vi "04. Streaming Simulator.vi"(8 "error in":errorcluster, 10 "request":T1, 11 "Actor Class":T2) -> (0 "error out":errorcluster)   [LabVIEW 2019]
uses:
  Actor/Actor Private Data.ctl
  <vilib>/LabVIEW Open Source Project/MQTT Client/Client class/Client.lvclass
  Actor/Actor Private Events -- cluster.ctl
  Actor/Payload -- cluster.ctl
  streaming-request -- cluster.ctl
  <vilib>/LabVIEW Open Source Project/OpenURI/uri/URI.lvclass/URI.ctl
  <vilib>/LabVIEW Open Source Project/OpenURI/uri/URI.lvclass
panel:
  out "Download Progress":dbl(slide) scale=0.0..100.0
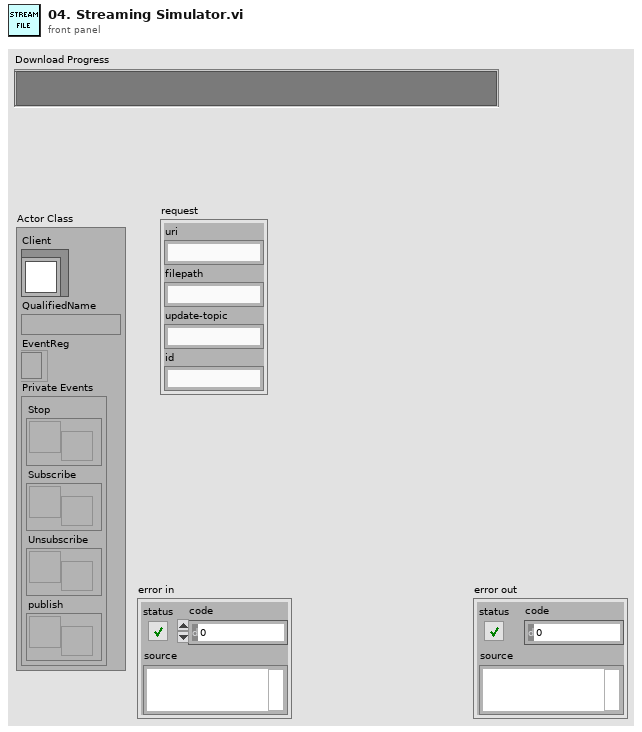
[diagram p1: front panel]
types:
  T1 = typedef "streaming-request -- cluster.ctl" = cluster{"uri":string, "filepath":string, "update-topic":string, "id":string}
  T2 = typedef "Actor Private Data.ctl" = cluster{"Client":refnum<class "Client.lvclass">, "QualifiedName":string, "EventReg":refnum<event-registration>, "Private Events":T3}
  T3 = typedef "Actor Private Events -- cluster.ctl" = cluster{"Stop":refnum<user-event>, "Subscribe":refnum<user-event>, "Unsubscribe":refnum<user-event>, "publish":refnum<user-event>}
  T4 = cluster{"progress (%)":dbl, "complete":bool, "error":bool}
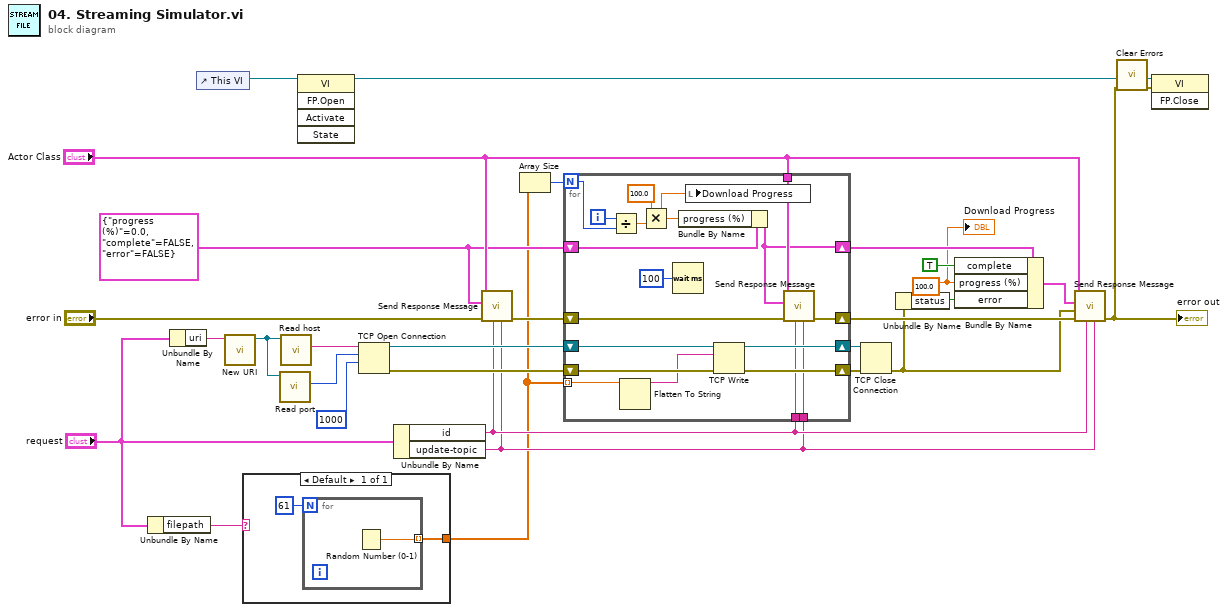
[diagram p0: block diagram]
diagram:
  w4 = 100.0 ("x")
  w26 = T4 {"progress (%)"=0.0, "complete"=FALSE, "error"=FALSE}
  n1 = Unbundle By Name("request") -> ("filepath"=w12:string)
  n2 = Unbundle By Name("request") -> ("uri"=w23:string)
  n3 = control-ref of="This VI"() -> (w5:refnum<vi>)
  n4 = call <vilib>:"New URI.vi"("URI"=w23) -> ("URI"=w21:refnum<class "URI.lvclass">)  [unwired: 9 in, 1 out]
  n5 = case shown="Default" w12 {
    tunnel: [w31] -> w10
    frame Default {
      n6 = for {
        N: 61 ("dimension size") -> [_]
        tunnel: [w33] -> w31 mode=indexing
        n7 = Random Number (0-1)() -> (number: 0 to 1=w33:dbl)
      }
    }
  }
  n8 = call <vilib>:"Read port.vi"("URI in"=w21) -> ("port"=w20:u16)  [unwired: 8 in, 2 out]
  n9 = call <vilib>:"Read host.vi"("URI in"=w21) -> ("host"=w22:string)  [unwired: 8 in, 2 out]
  n10 = invoke class="VI" method="FP.Open"(reference=w5) -> (reference out=w3:refnum<vi>)  [unwired: 4 in, 4 out]
  n11 = TCP Open Connection(address=w22, remote port or service name=w20, timeout ms (60000)=1000) -> (connection ID=w19:refnum<k5>, error out=w17:errorcluster)  [unwired: 2 in]
  n12 = Unbundle By Name("request") -> ("id"=w15:string, "update-topic"=w14:string)
  n13 = call "Send Response Message.vi"("topic"=w14, "id"=w15, "error in"="error in", "result"=w26, "Actor Class"="Actor Class") -> ("error out"=w28:errorcluster)  [unwired: 5 in, 1 out]
  n14 = Array Size(array=w10) -> (size(s)=w11:i32)
  n15 = for {
    N: w11 -> [w46]
    tunnel: "Actor Class" -> [w50]
    shift-right: [w51] -> w30
    shift-left: w28 -> [w52]
    shift-right: [w43] -> w25
    shift-left: w26 -> [w48]
    shift-right: [w39] -> w18
    shift-left: w19 -> [w40]
    shift-right: [w41] -> w16
    shift-left: w17 -> [w42]
    tunnel: w15 -> [w38]
    tunnel: w14 -> [w37]
    tunnel: w10 -> [w36] mode=indexing
    i -> [w47]
    n16 = Divide(x=w47, y=w46) -> (x/y=w45:dbl)
    n17 = Flatten To String(anything=w36) -> (data string=w35:string)  [unwired: 3 in, 2 out]
    n18 = Multiply(x=100.0, y=w45) -> (x*y=w34:dbl)
    n19 = Wait (ms)(milliseconds to wait=u32 100) -> ()  [unwired: 1 out]
    n20 = Bundle By Name(cluster=w48, "progress (%)"=w34) -> (w43:T4)
    n21 = local write "Download Progress"(w34) -> ()
    n22 = TCP Write(connection ID=w40, data in=w35, error in (no error)=w42) -> (connection ID out=w39:refnum<k5>, error out=w41:errorcluster)  [unwired: 1 in, 1 out]
    n23 = call "Send Response Message.vi"("topic"=w37, "id"=w38, "error in"=w52, "result"=w43, "Actor Class"=w50) -> ("error out"=w51:errorcluster)  [unwired: 5 in, 1 out]
  }
  n24 = TCP Close Connection(connection ID=w18, error in (no error)=w16) -> (error out=w7:errorcluster)  [unwired: 1 in, 1 out]
  n25 = Unbundle By Name(w7) -> ("status"=w6:bool)
  n26 = Bundle By Name(cluster=w25, "complete"=TRUE, "progress (%)"=w4, "error"=w6) -> (w8:T4)
  n27 = call "Send Response Message.vi"("topic"=w14, "id"=w15, "error in"=w30, "request error"=w7, "result"=w8, "Actor Class"="Actor Class") -> ("error out"=w2:errorcluster)  [unwired: 4 in, 1 out]
  "error out" <- w2
  n28 = call <vilib>:"Clear Errors.vi"("error in (no error)"=w2) -> ("error out"=w1:errorcluster)  [unwired: 5 in, 1 out]
  n29 = invoke class="VI" method="FP.Close"(reference=w3, error in=w1) -> ()  [unwired: 1 in, 3 out]
  "Download Progress" <- w4
